vi "ApplyCalibration.vi"(2 "Potentials":dbl[](array[numeric])=[-118.0, -100.0, -100.0, -100.0, -120.0, -120.0, -120.0, 0.0, 0.0, 0.0, 0.0, 0.0, 0.0, 0.0, 0.0, 10.0, 0.0, 0.0, 0.0, 0.0, 0.0, 0.0], 4 "# AO cards":u8=2, 5 "Calibrations":T1=[{"Gain"=15.0275, "Offset (V)"=0.0002, "Name"="U11"}, {"Gain"=15.032, "Offset (V)"=0.0002, "Name"="U10"}, {"Gain"=15.0677, "Offset (V)"=0.0002, "Name"="U9"}, {"Gain"=15.0236, "Offset (V)"=0.0001, "Name"="U8"}, {"Gain"=15.0405, "Offset (V)"=0.0001, "Name"="U7"}, {"Gain"=15.042, "Offset (V)"=0.0001, "Name"="U6"}, {"Gain"=15.0309, "Offset (V)"=0.0001, "Name"="U5"}, {"Gain"=15.0621, "Offset (V)"=0.0025, "Name"="U4"}, {"Gain"=15.0, "Offset (V)"=0.0, "Name"="U3"}, {"Gain"=15.0, "Offset (V)"=0.0, "Name"="U2"}, {"Gain"=15.0, "Offset (V)"=0.0, "Name"="U1"}, {"Gain"=15.0, "Offset (V)"=0.0, "Name"="D1"}, {"Gain"=15.0, "Offset (V)"=0.0, "Name"="D2"}, {"Gain"=15.0, "Offset (V)"=0.0, "Name"="D3"}, {"Gain"=15.0, "Offset (V)"=0.0, "Name"="D4"}, {"Gain"=15.0, "Offset (V)"=0.0, "Name"="mF"}] {"Offset (V)" format="%_6p"; "Gain" format="%_6p"}) -> (0 "# always zero":i32, 1 "Excitations":dbl[](array[numeric])=[-7.852284145732824, -6.6524880255455034, -6.63672624222675, -6.6562009105673745, -7.978464811675144, -7.977669192926473, -7.983560531970807, -0.0001659795114891018, 0.0, 0.0, 0.0, 0.0, 0.0, 0.0, 0.0, 0.6666666666666666])   [LabVIEW 2018]
uses:
  Calibrations.ctl
panel:
  out "#Potentials > #AO chans":bool=TRUE
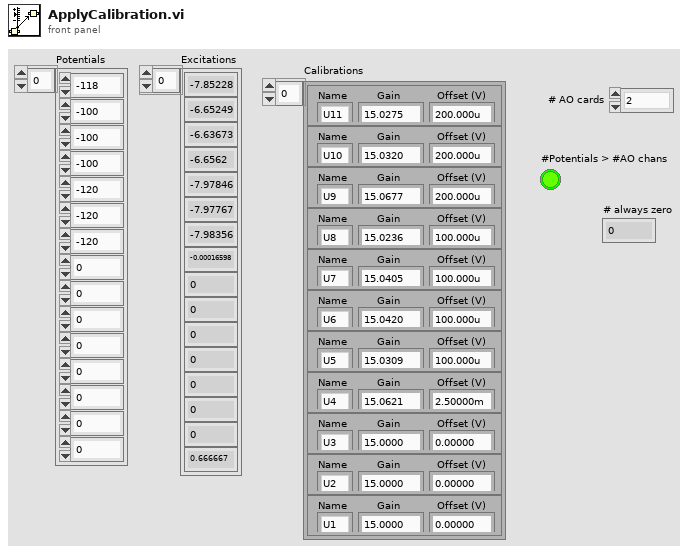
[diagram p1: front panel]
types:
  T1 = typedef "Calibrations.ctl" = cluster{"Gain":dbl, "Offset (V)":dbl, "Name":string}[]
  T2 = cluster{"Gain":dbl, "Offset (V)":dbl, "Name":string}
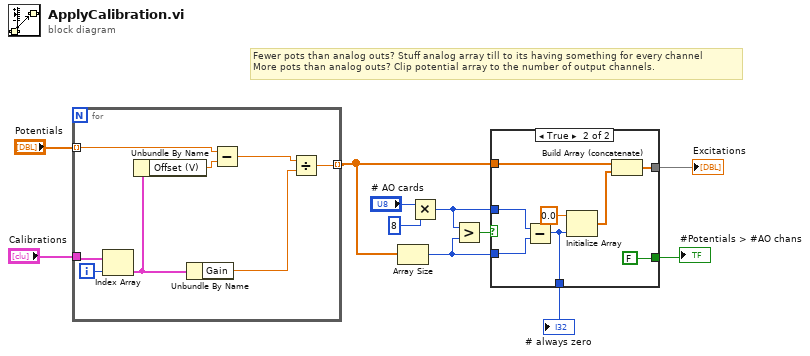
[diagram p0: block diagram]
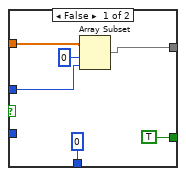
[diagram p2: hidden frame]
diagram:
  # "Fewer pots than analog outs? Stuff analog array till to its having something for every channel\nMore pots than analog outs? Clip potential array to the number of output channels."
  n1 = for {
    tunnel: "Calibrations" -> [w18]
    tunnel: "Potentials" -> [w15] mode=indexing
    tunnel: [w12] -> w5 mode=indexing
    i -> [w19]
    n2 = Index Array(array=w18, index=w19) -> (element=w17:T2)
    n3 = Unbundle By Name(w17) -> ("Offset (V)"=w16:dbl)
    n4 = Unbundle By Name(w17) -> ("Gain"=w13:dbl)
    n5 = Subtract(x=w15, y=w16) -> (x-y=w14:dbl)
    n6 = Divide(x=w14, y=w13) -> (x/y=w12:dbl)
  }
  n7 = Array Size(array=w5) -> (size(s)=w3:i32)
  n8 = Multiply(x="# AO cards", y=u8 8) -> (x*y=w4:u8)
  n9 = Greater?(x=w4, y=w3) -> (0:w2:bool)
  n10 = case shown="True" w2 {
    tunnel: [0 w33] -> w7
    tunnel: [w21 w30] -> w6
    tunnel: w5 -> [w24 w29]
    tunnel: w4 -> [w23 w28]
    tunnel: w3 -> [_ w27]
    tunnel: [TRUE ("#Potentials > #AO chans") FALSE ("#Potentials > #AO chans")] -> w1
    frame False {
      n11 = Array Subset(array=w24, index=0, length=w23) -> (w21:dbl[])
    }
    frame True {
      n12 = Subtract(x=w28, y=w27) -> (x-y=w33:i32)
      n13 = Initialize Array(0.0 ("element"), w33) -> (w31:dbl[])
      n14 = Build Array (concatenate)(w29, w31) -> (w30:dbl[])
    }
  }
  "Excitations" <- w6
  "# always zero" <- w7
  "#Potentials > #AO chans" <- w1
